vi "Status OSc.vi"(8 "error in (no error)":errorcluster, 10 "data":variant, 11 "Control-Client in":refnum<class "Control-Client.lvclass">) -> (0 "error out":errorcluster, 2 "error IO":errorcluster, 3 "Control-Client out":refnum<class "Control-Client.lvclass">)   [LabVIEW 2020, in "Control-Client.lvclass"]
uses:
  Control-Client.lvclass
  C:/dev/TRANCON/Classes/GeneralFunctionality/GeneralFunctionality.lvclass
  dependecies/ControlsVIs/Clusters-def/Commands-CLIENT.ctl
  dependecies/ControlsVIs/Clusters-def/Message types.ctl
  dependecies/ControlsVIs/Clusters-def/OSc-Reply-Connect-client.ctl
  Control-Client.lvclass/Control-Client.ctl
  controls/Gauge_pump/Gauge_pump.xctl
  dependecies/XControls/CellsDL/ControlDL.xctl
  Message/Message.lvclass
  GeneralFunctionality/GeneralFunctionality.lvclass
  Oscilloscope/Oscilloscope.lvclass
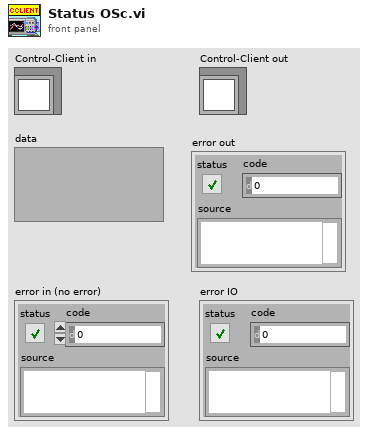
[diagram p1: front panel]
types:
  T1 = typedef "Oscilloscope.lvclass/OSc-Reply-Connect-Client.ctl" = cluster{"on/off":bool, "WCM_state":bool, "error":errorcluster}
  T2 = typedef "Message types.ctl" = string
  T3 = typedef "Control-Client.lvclass/Commands-CLIENT.ctl" = string
  T4 = typedef "Control-Client.lvclass/Controls-with-permissions_CLIENT.ctl" = cluster{"Server ON/OFF":refnum<vi>, "Detector connect":refnum<vi>, "DL connect":refnum<vi>, "DAQmx connect":refnum<vi>, "All connect":refnum<vi>, "Start measurement":refnum<vi>, "Move Crystal":refnum<vi>, "Relay key heater":refnum<vi>, "Laser Shutter":refnum<vi>, "Accelerator Shutter":refnum<vi>, "Power":refnum<vi>, "Unlock":refnum<vi>, "RT":refnum<vi>, "Faraday Cup":refnum<vi>, "Osc connect":refnum<vi>, "ELYSE pulses":refnum<vi>, "Cells":refnum<vi>, "Pump":refnum<vi>, "# par point":refnum<vi>, "Alarm":refnum<vi>, "oscilloscopeRead":refnum<vi>, "WCM_state":refnum<vi>, "ControlDL":refnum<vi>}
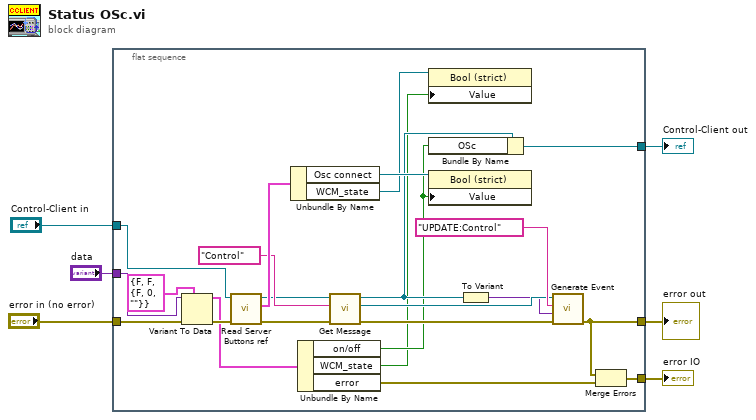
[diagram p0: block diagram]
diagram:
  n1 = flat-sequence {
    tunnel: "data" -> [w29]
    tunnel: "Control-Client in" -> [w28]
    tunnel: "error in (no error)" -> [w26]
    tunnel: [w10] -> w5
    tunnel: [w15] -> w6
    tunnel: [w11] -> w1
    frame #0 {
      n2 = Variant To Data(error in=w26, type=T1 {"on/off"=FALSE, "WCM_state"=FALSE, "error"={"status"=FALSE, "code"=0, "source"=""}} ("output cluster"), Variant=w29) -> (data=w16:T1, error out=w27:errorcluster)
      n3 = call "Read Server Buttons ref.vi"("error in (no error)"=w27, "Control-Client in"=w28) -> ("error out"=w17:errorcluster, "Server Buttons ref"=w25:T4, "Control-Client out"=w18:refnum<class "Control-Client.lvclass">)  [unwired: 7 in]
      n4 = Unbundle By Name(w25) -> ("Osc connect"=w24:refnum<vi>, "WCM_state"=w8:refnum<vi>)
      n5 = Unbundle By Name(w16) -> ("on/off"=w9:bool, "WCM_state"=w7:bool, "error"=w12:errorcluster)
      n6 = call "Get Message.vi"("error in (no error)"=w17, "Message type"=T2 "Control", "GeneralFunctionality en entrée"=w18) -> ("error out"=w20:errorcluster, "Message.lvclass"=w22:refnum<class "Message.lvclass">, "GeneralFunctionality en sortie"=w14:refnum<class "Control-Client.lvclass">)  [unwired: 6 in]
      n7 = property class="Bool (strict)"(reference=w8, "Value"=w7) -> ()  [unwired: 1 in, 2 out]
      n8 = Bundle By Name(cluster=w14, "OSc"=w9) -> (w10:refnum<class "Control-Client.lvclass">)
      n9 = property class="Bool (strict)"(reference=w24, "Value"=w9) -> ()  [unwired: 1 in, 2 out]
      n10 = To Variant(anything=w14) -> (Variant=w19:variant)
      n11 = call "Generate Event.vi"("error in (no error)"=w20, "Data"=w19, "Command"=T3 "UPDATE:Control" ("Commands-Client"), "Message en entrée"=w22) -> ("error out"=w11:errorcluster)  [unwired: 6 in, 1 out]
      n12 = Merge Errors(w11, w12) -> (w15:errorcluster)
    }
  }
  "error IO" <- w6
  "Control-Client out" <- w5
  "error out" <- w1
